vi "Get Available Templates.vi"(8 "error in (no error)":errorcluster) -> (0 "error out":errorcluster, 3 "Templates":T1[](array[typedef]))   [LabVIEW 2013, in "Project Wizard.lvlib"]
uses:
  Project Wizard.lvlib
  controls/Template.ctl
  <vilib>/Utility/sysdir.llb/System Directory Type.ctl
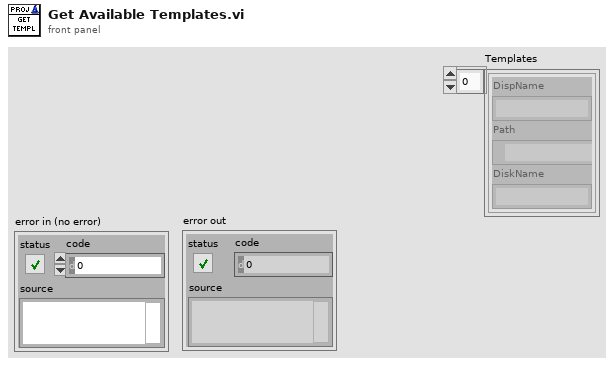
[diagram p1: front panel]
types:
  T1 = typedef "Project Wizard.lvlib/Template.ctl" = cluster{"DispName":string, "Path":path, "DiskName":string}
  T2 = typedef "System Directory Type.ctl" = i32
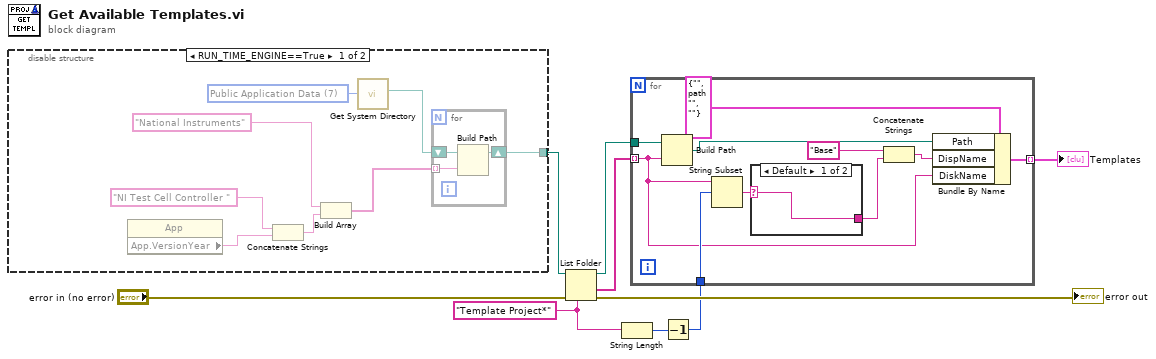
[diagram p0: block diagram]
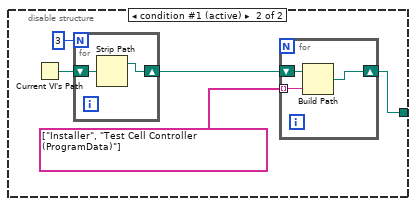
[diagram p3: hidden frame]
diagram:
  w3 = "Template Project*" ("pattern")
  n1 = disable-structure shown="RUN_TIME_ENGINE==True" {
    disable-tunnel: [w15 w21] -> w6
    frame condition #0 {
      w17 = T2 7 items=["User Home"=0, "User Desktop"=1, "User Documents"=2, "User Application Data"=3, "User Preferences"=4, "User Temporary"=5, "Public Documents"=6, "Public Application Data"=7, "Public Preferences"=8, "Public Cache"=13, "System Core Libraries"=9, "System Installed Libraries"=10, "Application Files"=11, "Boot Volume Root"=12] ("system directory type")
      n2 = property class="App"() -> ("App.VersionYear"=w14:string)  [unwired: 2 in, 2 out]
      n3 = Concatenate Strings("NI Test Cell Controller " ("name or relative path"), w14) -> (w12:string)
      n4 = Build Array("National Instruments" ("name or relative path"), w12) -> (w10:string[])
      n5 = call <vilib>:"Get System Directory.vi"("system directory type"=w17) -> ("system directory"=w16:path)  [unwired: 10 in]
      n6 = for {
        tunnel: w10 -> [w19] mode=indexing
        shift-right: [w20] -> w15
        shift-left: w16 -> [w18]
        n7 = Build Path(base path=w18, name or relative path=w19) -> (appended path=w20:path)
      }
    }
    frame condition #1 (active) {
      n8 = Current VI's Path() -> (path=w25:path)
      n9 = for {
        N: 3 -> [_]
        shift-right: [w29] -> w23
        shift-left: w25 -> [w30]
        n10 = Strip Path(path=w30) -> (stripped path=w29:path)  [unwired: 1 out]
      }
      n11 = for {
        shift-right: [w27] -> w21
        shift-left: w23 -> [w28]
        tunnel: string[] ["Installer", "Test Cell Controller (ProgramData)"] -> [w26] mode=indexing
        n12 = Build Path(base path=w28, name or relative path=w26) -> (appended path=w27:path)
      }
    }
  }
  n13 = List Folder(path=w6, pattern=w3, error in="error in (no error)") -> (path out=w4:path, folder names=w5:string[], error out=→"error out":errorcluster)  [unwired: 1 in, 1 out]
  n14 = String Length(string=w3) -> (length=w2:i32)
  n15 = Decrement(x=w2) -> (x-1=w1:i32)
  n16 = for {
    tunnel: w5 -> [w31] mode=indexing
    tunnel: w4 -> [w39]
    tunnel: [w37] -> w7 mode=indexing
    tunnel: w1 -> [w36]
    n17 = Build Path(base path=w39, name or relative path=w31) -> (appended path=w38:path)
    n18 = String Subset(string=w31, offset (0)=w36) -> (substring=w35:string)  [unwired: 1 in]
    n19 = case shown="Default" w35 {
      selector: w35 -> [w41 _]
      tunnel: [w41 _] -> w32
      frame Default {
      }
      frame "" {
      }
    }
    n20 = Concatenate Strings("Base", w32) -> (w33:string)
    n21 = Bundle By Name(cluster=T1 {"DispName"="", "Path"=path "", "DiskName"=""} ("Template"), "Path"=w38, "DispName"=w33, "DiskName"=w31) -> (w37:T1)
  }
  "Templates" <- w7
